vi "const exceptioncausename.vi"() -> (3 "label":string)   [LabVIEW 2013, in "exception.lvlib"]
uses:
  exception.lvlib
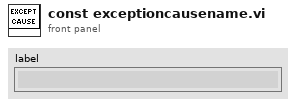
[diagram p1: front panel]
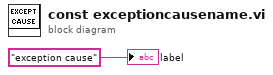
[diagram p0: block diagram]
diagram:
  "label" <- "exception cause"
